vi "Practica_3.vi"() -> ()   [LabVIEW 2022 SP3]
uses:
  <vilib>/Utility/NIReport.llb/Report Type.ctl
  <vilib>/imath/engines/lvmath2/RunTimeEngine/Managers/WorkSpace/UID Generator.vi
  <vilib>/imath/engines/lvmath2/RunTimeEngine/RunTimeType/NIMS_RunTimeType_From StrictType (excl LVString).vi
  <instcachedir>/0/NIMS_RunTimeType_From StrictType (excl LVString)_70DEE8F51B6B495C85F505DE4E7061F1.lvgen/NIMS_RunTimeType_From StrictType (excl LVString)_70DEE8F51B6B495C85F505DE4E7061F1_000.vi
  <vilib>/imath/engines/lvmath2/RunTimeEngine/LocalVariableDefStatement/MC_LocalVariableDefStatement_Display.vi
  <vilib>/imath/engines/lvmath2/RunTimeEngine/VariableToken/NIMS_VariableToken_CondDefined.vi
  <instcachedir>/0/NIMS_VariableToken_CondDefined_190C34D11DD44198A50DB545329B6163.lvgen/NIMS_VariableToken_CondDefined_190C34D11DD44198A50DB545329B6163_003.vi
  <vilib>/imath/engines/lvmath2/RunTimeEngine/BuiltInFunctions/tf_to_ss/NIMS_tf_to_ss.vi
  <vilib>/imath/engines/lvmath2/RunTimeEngine/ErrorHandling/NIMS_Create Error From Enums.vi
  <vilib>/imath/engines/lvmath2/RunTimeEngine/BuiltInFunctions/transpose/NIMS_transpose(GM).vi
  <instcachedir>/0/NIMS_transpose(GM)_822C4B39CC3F4B34B360A85316D387F1.lvgen/NIMS_transpose(GM)_822C4B39CC3F4B34B360A85316D387F1_004.vi
  <vilib>/imath/engines/lvmath/Plug In/Control Design/BuiltInFunctions/obsvmx/NIMS_CD_obsvmx(A,B).vi
  <vilib>/imath/engines/lvmath/Plug In/Control Design/BuiltInFunctions/ctrbmx/NIMS_CD_ctrbmx(A,B).vi
  <vilib>/imath/engines/lvmath2/RunTimeEngine/BuiltInFunctions/rank/NIMS_rank.vi
  <instcachedir>/0/NIMS_rank_39A1B4AED7134F5694149EE328E336E6.lvgen/NIMS_rank_39A1B4AED7134F5694149EE328E336E6_000.vi
  <vilib>/imath/engines/lvmath2/RunTimeEngine/ErrorHandling/NIMS_Error From Error Code.vi
  <vilib>/imath/engines/lvmath2/RunTimeEngine/BuiltInFunctions/det/NIMS_det.vi
  <instcachedir>/0/NIMS_det_FC43403F6A814B2FA6A2876A6DC65E99.lvgen/NIMS_det_FC43403F6A814B2FA6A2876A6DC65E99_000.vi
  <vilib>/imath/engines/lvmath/Plug In/Control Design/BuiltInFunctions/ss/NIMS_CD_ss(A,B,C,D).vi
  <instcachedir>/0/NIMS_RunTimeType_From StrictType (excl LVString)_70DEE8F51B6B495C85F505DE4E7061F1.lvgen/NIMS_RunTimeType_From StrictType (excl LVString)_70DEE8F51B6B495C85F505DE4E7061F1_032.vi
  <vilib>/imath/engines/lvmath/Plug In/Control Design/BuiltInFunctions/step/NIMS_CD_[Y,T,X]=step(SS,[Tinfo]).vi
  <vilib>/imath/engines/lvmath2/RunTimeEngine/BuiltInFunctions/inv/NIMS_inv(GM).vi
  <instcachedir>/0/NIMS_inv(GM)_A6DF8FE880224208AACFE4CF9F659502.lvgen/NIMS_inv(GM)_A6DF8FE880224208AACFE4CF9F659502_000.vi
  <vilib>/imath/engines/lvmath2/RunTimeEngine/BuiltInFunctions/size/NIMS_I32Row=size(GM).vi
  <instcachedir>/0/NIMS_I32Row=size(GM)_10ACDCB9F1F84A7E9F42C91D87611FB5.lvgen/NIMS_I32Row=size(GM)_10ACDCB9F1F84A7E9F42C91D87611FB5_001.vi
  <vilib>/imath/engines/lvmath2/RunTimeEngine/IndexRead/NIMS V(S).vi
  <instcachedir>/0/NIMS V(S)_0488751826AF41519A22953C041130DC.lvgen/NIMS V(S)_0488751826AF41519A22953C041130DC_002.vi
  <vilib>/imathl/engines/lvmath/Functions/Error Handling/Create Error.vi
  <instcachedir>/0/NIMS_VariableToken_CondDefined_190C34D11DD44198A50DB545329B6163.lvgen/NIMS_VariableToken_CondDefined_190C34D11DD44198A50DB545329B6163_001.vi
  <instcachedir>/0/NIMS_VariableToken_CondDefined_190C34D11DD44198A50DB545329B6163.lvgen/NIMS_VariableToken_CondDefined_190C34D11DD44198A50DB545329B6163_005.vi
  <instcachedir>/0/NIMS_VariableToken_CondDefined_190C34D11DD44198A50DB545329B6163.lvgen/NIMS_VariableToken_CondDefined_190C34D11DD44198A50DB545329B6163_004.vi
  <vilib>/imath/engines/lvmath/Functions/Error Handling/MergeErrorsWrapper.vi
  <vilib>/imath/engines/lvmath2/RunTimeEngine/Managers/SymbolTable/Clear UID.vi
  <vilib>/imath/engines/lvmath2/RunTimeEngine/NodeEndStatement/NIMS_NodeEndStatement_Output.vi
  <instcachedir>/0/NIMS_NodeEndStatement_Output_53EC0D466D134D7ABD903AC30B43404B.lvgen/NIMS_NodeEndStatement_Output_53EC0D466D134D7ABD903AC30B43404B_009.vi
  <instcachedir>/0/NIMS_NodeEndStatement_Output_53EC0D466D134D7ABD903AC30B43404B.lvgen/NIMS_NodeEndStatement_Output_53EC0D466D134D7ABD903AC30B43404B_002.vi
  <instcachedir>/0/NIMS_NodeEndStatement_Output_53EC0D466D134D7ABD903AC30B43404B.lvgen/NIMS_NodeEndStatement_Output_53EC0D466D134D7ABD903AC30B43404B_001.vi
  <vilib>/imath/engines/lvmath2/RunTimeEngine/ErrorHandling/NIMS_Finalize Error.vi
  <vilib>/imath/engines/lvmath2/RunTimeEngine/BuiltInFunctions/sin/NIMS_sin(C).vi
  <instcachedir>/0/NIMS_sin(C)_E954A9BB68A349B3841053E554BADAA4.lvgen/NIMS_sin(C)_E954A9BB68A349B3841053E554BADAA4_001.vi
  <vilib>/imath/engines/lvmath2/RunTimeEngine/BuiltInFunctions/cos/NIMS_cos(C).vi
  <instcachedir>/0/NIMS_cos(C)_24E28D29219C4DC6ABC084DC6A0254BF.lvgen/NIMS_cos(C)_24E28D29219C4DC6ABC084DC6A0254BF_001.vi
  <vilib>/imath/engines/lvmath2/RunTimeEngine/BuiltInFunctions/length/NIMS_length(GM).vi
  <instcachedir>/0/NIMS_length(GM)_47CEC356FCE0482D9BA47DC61C99F2C7.lvgen/NIMS_length(GM)_47CEC356FCE0482D9BA47DC61C99F2C7_000.vi
  <vilib>/imath/engines/lvmath2/RunTimeEngine/BuiltInFunctions/zeros/NIMS_V=zeros(I32,I32).vi
  <vilib>/imath/engines/lvmath2/RunTimeEngine/RowToken/NIMS_RowToken_M_M.vi
  <instcachedir>/0/NIMS_RowToken_M_M_4BA134D7580D4B93A915AC56DC6FEFD1.lvgen/NIMS_RowToken_M_M_4BA134D7580D4B93A915AC56DC6FEFD1_004.vi
  <vilib>/imath/engines/lvmath2/RunTimeEngine/MatrixToken/NIMS_MatrixToken_M_RV.vi
  <instcachedir>/0/NIMS_MatrixToken_M_RV_FA177D3434DD41A3B3A5813DE937EEA2.lvgen/NIMS_MatrixToken_M_RV_FA177D3434DD41A3B3A5813DE937EEA2_001.vi
  <vilib>/imath/engines/lvmath/Plug In/Control Design/BuiltInFunctions/ackermann/NIMS_CD_ackermann(A,B,poles,STR).vi
  <vilib>/imath/engines/lvmath2/RunTimeEngine/BuiltInFunctions/eye/NIMS_M=eye(I32).vi
  <vilib>/imath/engines/lvmath2/RunTimeEngine/ArithmeticOperatorToken/NIMS_ArithmeticOperator_minus.vi
  <instcachedir>/0/NIMS_ArithmeticOperator_minus_22EE3FD1C8824638A4ED1C446A3DB56D.lvgen/NIMS_ArithmeticOperator_minus_22EE3FD1C8824638A4ED1C446A3DB56D_001.vi
  <vilib>/imath/engines/lvmath2/RunTimeEngine/ArithmeticOperatorToken/NIMS_ArithmeticOperator_plus.vi
  <instcachedir>/0/NIMS_ArithmeticOperator_plus_3E2F46F6B6A2434E909AF418D4802C21.lvgen/NIMS_ArithmeticOperator_plus_3E2F46F6B6A2434E909AF418D4802C21_011.vi
  <vilib>/imath/engines/lvmath2/RunTimeEngine/ArithmeticOperatorToken/NIMS_ArithmeticOperator_multmx.vi
  <instcachedir>/0/NIMS_ArithmeticOperator_multmx_BDE1B5075EB4429787EED704427CBD98.lvgen/NIMS_ArithmeticOperator_multmx_BDE1B5075EB4429787EED704427CBD98_004.vi
  <vilib>/imath/engines/lvmath2/RunTimeEngine/MatrixToken/NIMS_MatrixToken_M_M.vi
  <instcachedir>/0/NIMS_MatrixToken_M_M_35B6F7FCE524444C982F4243CAF19F60.lvgen/NIMS_MatrixToken_M_M_35B6F7FCE524444C982F4243CAF19F60_004.vi
  <vilib>/imath/engines/lvmath2/RunTimeEngine/ArithmeticOperatorToken/NIMS_ArithmeticOperator_multmx(RV,M).vi
  <instcachedir>/0/NIMS_ArithmeticOperator_multmx(RV,M)_0C5EC56C64A44F5D9A149E640905A95E.lvgen/NIMS_ArithmeticOperator_multmx(RV,M)_0C5EC56C64A44F5D9A149E640905A95E_001.vi
  <vilib>/imath/engines/lvmath2/RunTimeEngine/IndexRead/NIMS M(R2).vi
  <instcachedir>/0/NIMS M(R2)_287818D58BD74005B29FE73CE7602B1A.lvgen/NIMS M(R2)_287818D58BD74005B29FE73CE7602B1A_000.vi
  <vilib>/imath/engines/lvmath2/RunTimeEngine/IndexRead/NIMS M(V).vi
  <instcachedir>/0/NIMS M(V)_948FAC22C1C943948B75DA6190348614.lvgen/NIMS M(V)_948FAC22C1C943948B75DA6190348614_005.vi
  <instcachedir>/0/NIMS_NodeEndStatement_Output_53EC0D466D134D7ABD903AC30B43404B.lvgen/NIMS_NodeEndStatement_Output_53EC0D466D134D7ABD903AC30B43404B_005.vi
  <instcachedir>/0/NIMS_NodeEndStatement_Output_53EC0D466D134D7ABD903AC30B43404B.lvgen/NIMS_NodeEndStatement_Output_53EC0D466D134D7ABD903AC30B43404B_008.vi
  <vilib>/imath/engines/lvmath2/RunTimeEngine/IndexRead/NIMS V($).vi
  <instcachedir>/0/NIMS V($)_C593F32C7F6B43C7B1793952E292524F.lvgen/NIMS V($)_C593F32C7F6B43C7B1793952E292524F_001.vi
  <vilib>/imath/engines/lvmath2/RunTimeEngine/ArithmeticOperatorToken/NIMS_ArithmeticOperator_multmx(M,CV).vi
  <instcachedir>/0/NIMS_ArithmeticOperator_multmx(M,CV)_F5DBFFF0126A4383B39F7B34D5ABA6C8.lvgen/NIMS_ArithmeticOperator_multmx(M,CV)_F5DBFFF0126A4383B39F7B34D5ABA6C8_000.vi
  <instcachedir>/0/NIMS_ArithmeticOperator_minus_22EE3FD1C8824638A4ED1C446A3DB56D.lvgen/NIMS_ArithmeticOperator_minus_22EE3FD1C8824638A4ED1C446A3DB56D_002.vi
  <vilib>/imath/engines/lvmath2/RunTimeEngine/IndexRead/NIMS M(S,S).vi
  <instcachedir>/0/NIMS M(S,S)_AC51E74150A542F7991B9634C66F3096.lvgen/NIMS M(S,S)_AC51E74150A542F7991B9634C66F3096_000.vi
  <vilib>/imath/engines/lvmath2/RunTimeEngine/IndexRead/NIMS M($).vi
  <instcachedir>/0/NIMS M($)_82D1177398184AFB96A6AFB63C3C3F57.lvgen/NIMS M($)_82D1177398184AFB96A6AFB63C3C3F57_000.vi
  <instcachedir>/0/NIMS_ArithmeticOperator_plus_3E2F46F6B6A2434E909AF418D4802C21.lvgen/NIMS_ArithmeticOperator_plus_3E2F46F6B6A2434E909AF418D4802C21_003.vi
  <vilib>/addons/_office/excel.llb/Excel Easy Table (num).vi
  <vilib>/Utility/NIReport.llb/NI_report.lvclass
  <vilib>/imath/engines/lvmath2/RunTimeEngine/Managers/SymbolTable/NIMS_WorkSpace.lvlib
  <vilib>/addons/_office/NI_ReportGenerationToolkit.lvlib
  <vilib>/Utility/NIReport.llb/Excel/NI_Excel.lvclass
  <vilib>/Utility/NIReport.llb/NI_ReportGenerationCore.lvlib
panel:
  out "xk1":dbl[](array[numeric])
  out "yk 2":dbl
  out "salida controlada":dbl
  out "set point":dbl
  in  "Tab Control":T1(tab)
  out "Observabilidad":string="El Sistema es Controlabe"
  out "Controlabilidas":string="El Sistema es Controlabe"
  out "Ta_Mo":i32
  out "Ta_Mc":i32
  out "GRAFICA":dbl[][](graph)
  out "Dete_MO":dbl
  out "Dete_MC":dbl
  out "Rango_MO":i32
  out "Rango_MC":i32
  out "MC":dbl[][](array[numeric])
  out "MO":dbl[][](array[numeric])
  out "CO":dbl[][](array[numeric])
  out "BO":dbl[][](array[numeric])
  out "AO":dbl[][](array[numeric])
  out "C":dbl[][](array[numeric])
  out "B":dbl[][](array[numeric])
  out "A":dbl[][](array[numeric])
  in  "ORDEN":dbl
  in  "Stop":bool
  in  "b4":dbl
  in  "a4":dbl
  in  "b3":dbl
  in  "a2":dbl
  in  "b2":dbl
  in  "b1":dbl
  in  "b0":dbl
  in  "a1":dbl
  in  "a3":dbl
  in  "tso":dbl
  in  "T":dbl
  in  "tss":dbl
  in  "Fa":dbl
  out "p1_o":cdb
  out "p2_o":cdb
  out "p1":cdb
  out "p2":cdb
  out "Ki":dbl[][](array[numeric])
  out "ks":dbl[][](array[numeric])
  out "L":dbl[](array[numeric])
  out "k1":dbl[][](array[numeric])
  in  "Sp":dbl
  out "Waveform Chart":T2(graph)
  out "error":dbl
  out "ley de control":dbl
  out "yk":dbl
  in  "template (empty)":path
  out "K":dbl[](array[numeric])
  out "0bservador":dbl
  # "z^-1  +"
  # "z^-2  +"
  # "z^-3  +"
  # "z^-4"
  # "+"
  # "Y(z)"
  # "G(Z)="
  # "="
  # "U(z)"
  # "z^-1  +"
  # "z^-2  +"
  # "z^-3  +"
  # "z^-4"
  # "1  +"
  # "FORMA CANONICA CONTROLABLE"
  # "FORMA CANONICA OBSERVABLE"
  # "CONTROLABILIDAD Y OBSERVABILIDAD DEL SISTEMA"
  # "CONDICIONES DE DISEÑO"
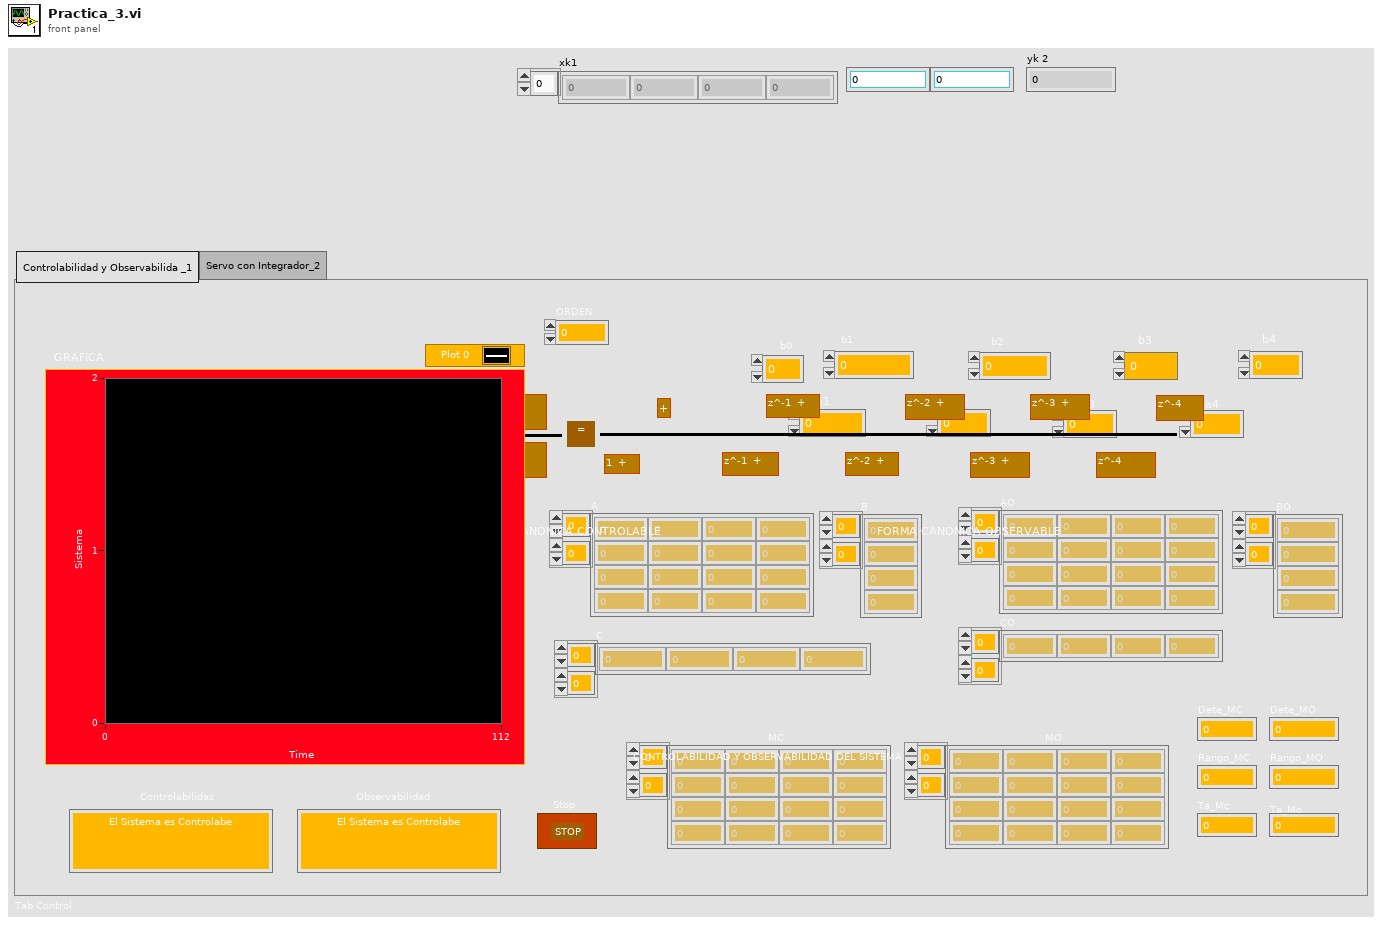
[diagram p1: front panel]
types:
  T1 = enum32{"Controlabilidad y Observabilida _1", "Servo con Integrador_2"}
  T2 = cluster{"yk":dbl, "Set-point":dbl, "error":dbl, dbl, dbl}
  T3 = typedef "NI_ReportGenerationCore.lvlib/Report Type.ctl" = enum16{"HTML", "Word", "Excel"}
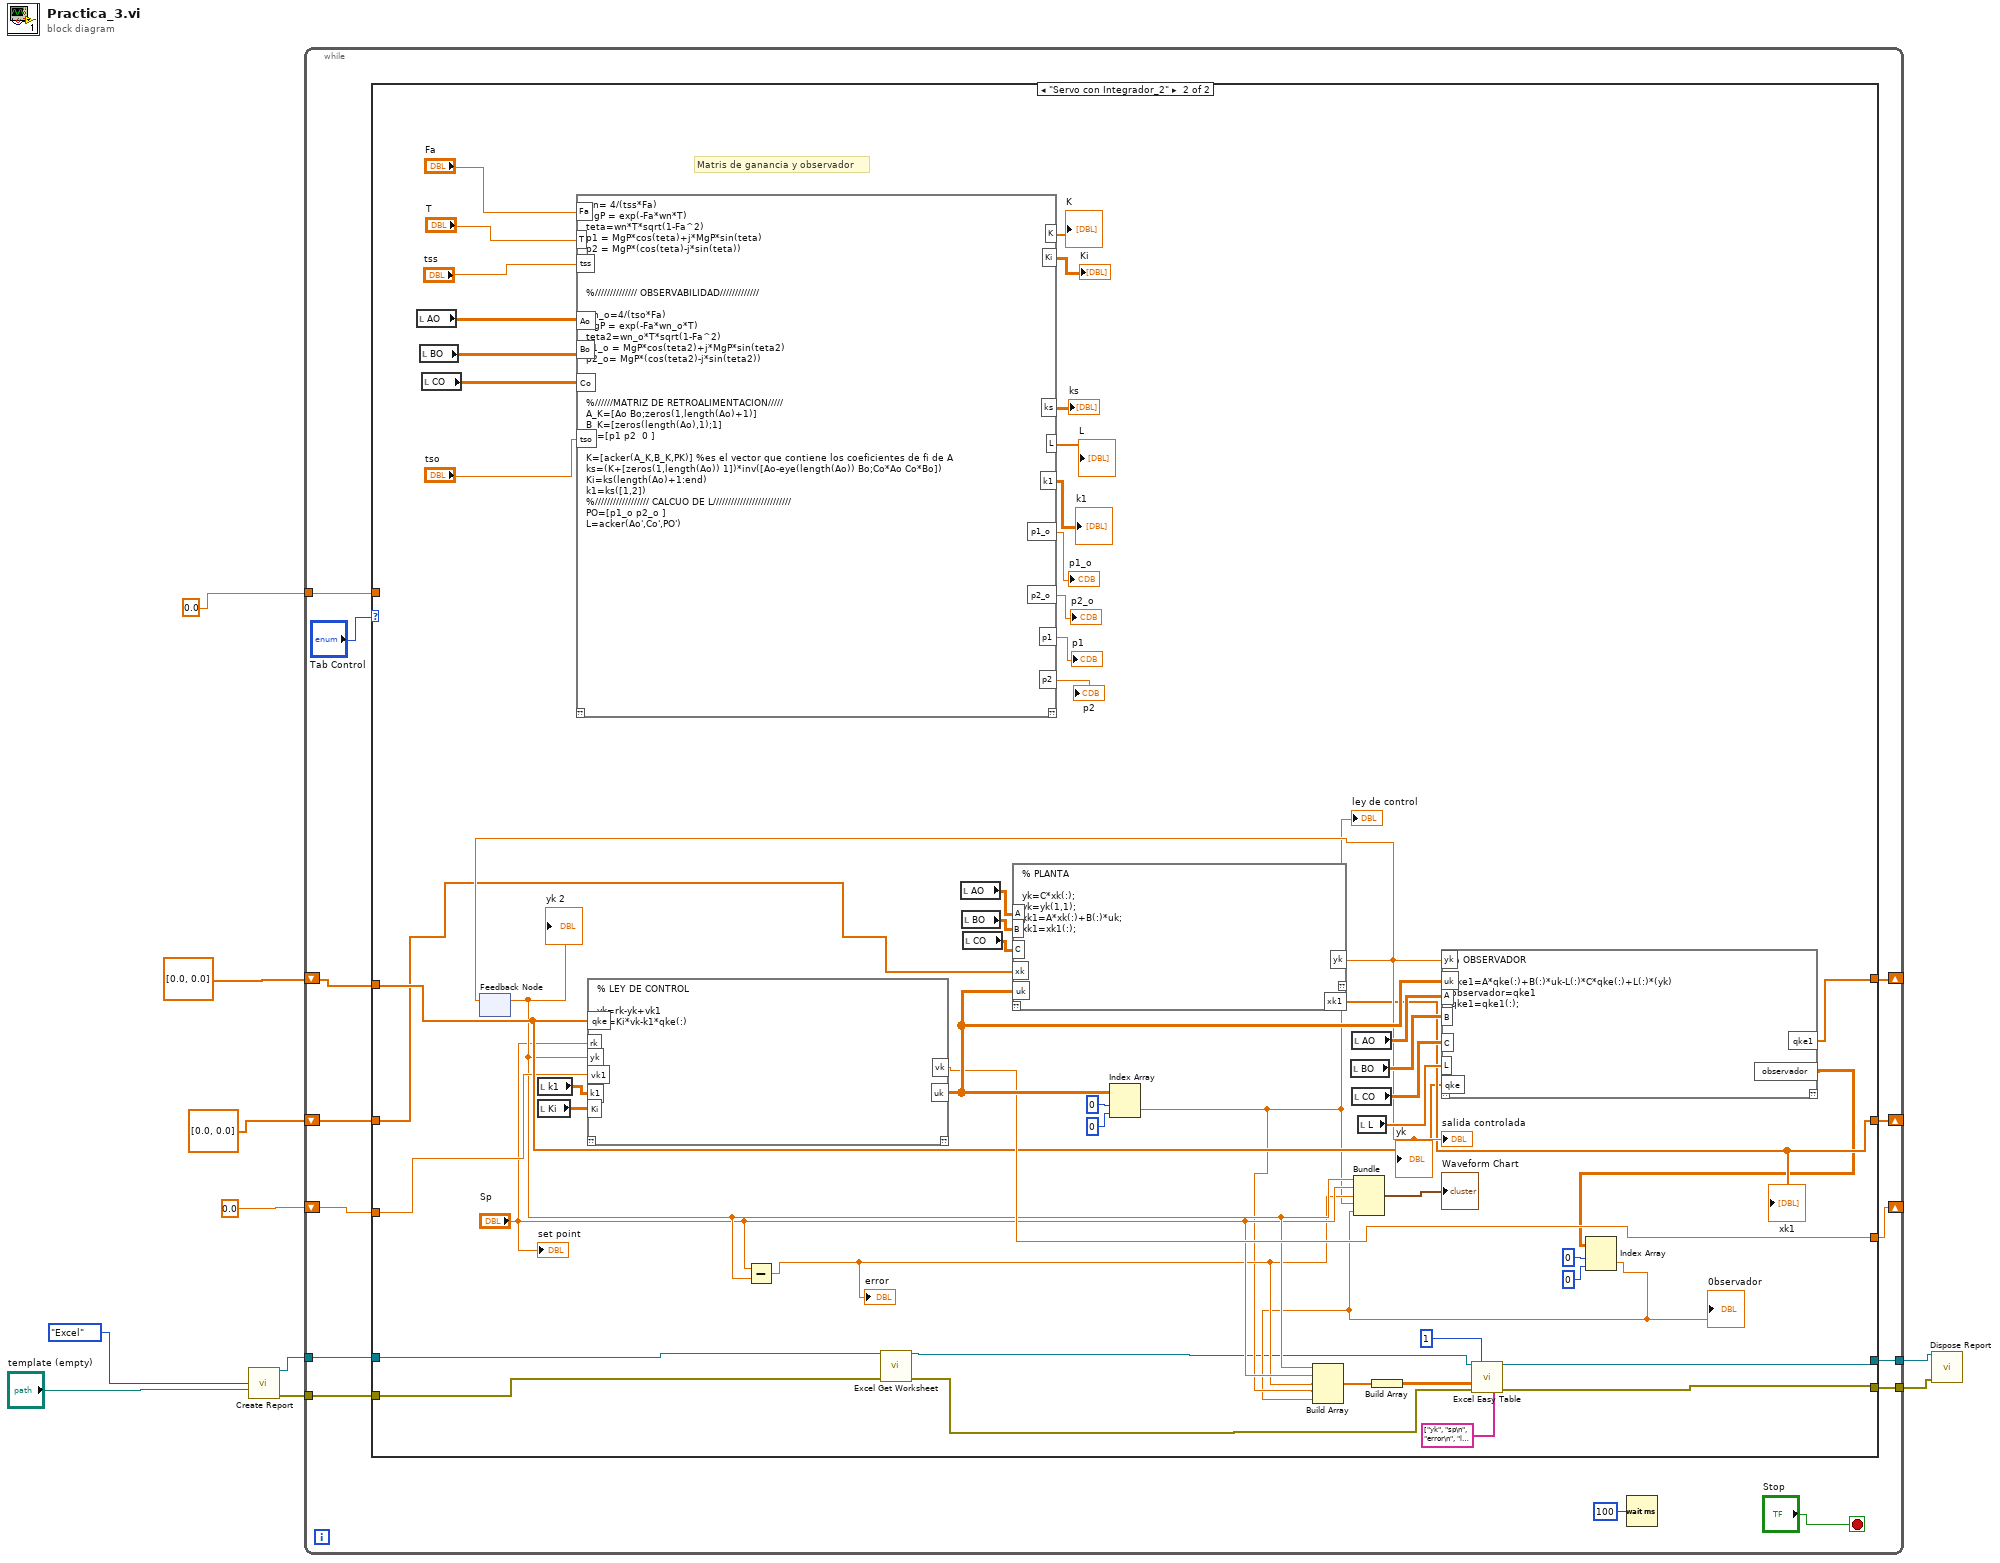
[diagram p0: block diagram]
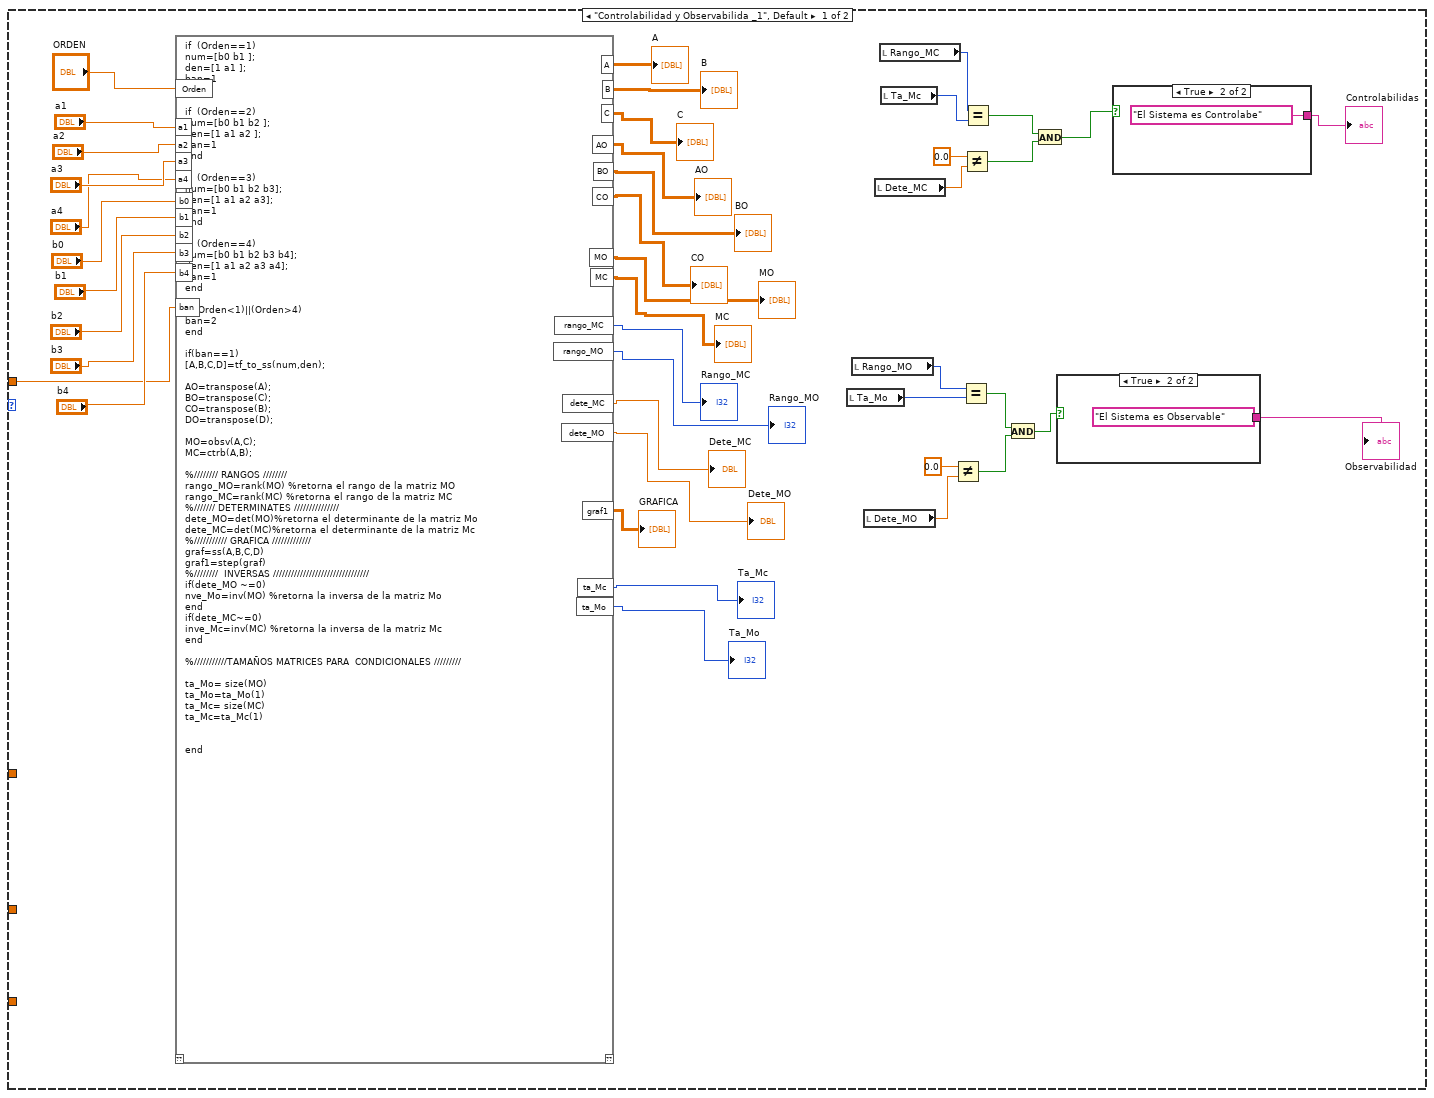
[diagram p2: hidden frame]
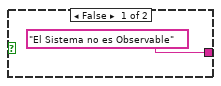
[diagram p3: hidden frame]
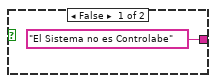
[diagram p4: hidden frame]
diagram:
  n1 = call <vilib>:"Create Report.vi"("report type"=Report_Type."Excel", "template (empty)"="template (empty)") -> ("report out"=w2:refnum<class "NI_report.lvclass">, "error out"=w1:errorcluster)  [unwired: 12 in]
  n2 = while {
    tunnel: 0.0 ("ban") -> [w22]
    shift-right: [w20] -> _
    shift-left: dbl[] [0.0, 0.0] ("qke1") -> [w19]
    shift-right: [w18] -> _
    shift-left: dbl[] [0.0, 0.0] ("xk1") -> [w17]
    shift-right: [w16] -> _
    shift-left: 0.0 ("yk") -> [w15]
    tunnel: [w14] -> w6
    tunnel: [w13] -> w5
    tunnel: w2 -> [w12]
    tunnel: w1 -> [w11]
    stop <- "Stop" stop-if-true
    n3 = case shown="\"Servo con Integrador_2\"" "Tab Control" {
      tunnel: w22 -> [w56 _]
      tunnel: [_ w1020] -> w20
      tunnel: w19 -> [_ w1016]
      tunnel: [_ w1019] -> w18
      tunnel: w17 -> [_ w1014]
      tunnel: [_ w1018] -> w16
      tunnel: w15 -> [_ w1015]
      tunnel: [_ w1002] -> w14
      tunnel: [_ w1001] -> w13
      tunnel: w12 -> [_ w1000]
      tunnel: w11 -> [_ w999]
      frame "Controlabilidad y Observabilida _1", Default {
        n4 = mathscript code="if  (Orden==1)\nnum=[b0 b1 ];\nden=[1 a1 ];\nban=1\nend \n\nif  (Orden==2)\nnum=[b0 b1 b2 ];\nden=[1 a1 a2 ];\nban=1\nend \n\nif  (Orden==3)\nnum=[b0 b1 b2 b3];\nden=[1 a1 a2 a3];\nban=1\nend \n\nif  (Orden==4)\nnum=[b0 b1 b2 b3 b4];\nden=[1 a1 a2 a3 a4];\nban=1\nend \n\nif (Orden<1)||(Orden>4)\nban=2\nend\n\nif(ban==1) \n[A,B,C,D]=tf_to_ss(num,den);\n\nAO=transpose(A);\nBO=transpose(C);\nCO=transpose(B);\nDO=transpose(D);\n\nMO=obsv(A,C);\nMC=ctrb(A,B);\n\n%//////// RANGOS ////////\nrango_MO=rank(MO) %retorna el rango de la matriz MO\nrango_MC=rank(MC) %retorna el rango de la matriz MC\n%/////// DETERMINATES ///////////////\ndete_MO=det(MO)%retorna el determinante de la matriz Mo\ndete_MC=det(MC)%retorna el determinante de la matriz Mc\n%/////////// GRAFICA /////////////\ngraf=ss(A,B,C,D)\ngraf1=step(graf)\n%////////  INVERSAS ////////////////////////////////\nif(dete_MO ~=0)\nnve_Mo=inv(MO) %retorna la inversa de la matriz Mo\nend\nif(dete_MC~=0)\ninve_Mc=inv(MC) %retorna la inversa de la matriz Mc\nend\n\n%///////////TAMAÑOS MATRICES PARA  CONDICIONALES /////////\n\nta_Mo= size(MO)\nta_Mo=ta_Mo(1)\nta_Mc= size(MC)\nta_Mc=ta_Mc(1)\n\n \nend"("a1"="a1", "a2"="a2", "a3"="a3", "a4"="a4", "b0"="b0", "b1"="b1", "b2"="b2", "b3"="b3", "b4"="b4", "Orden"="ORDEN", "ban"=w56) -> ("A"=→"A":dbl[][], "B"=→"B":dbl[][], "C"=→"C":dbl[][], "AO"=→"AO":dbl[][], "BO"=→"BO":dbl[][], "CO"=→"CO":dbl[][], "MO"=→"MO":dbl[][], "MC"=→"MC":dbl[][], "rango_MC"=→"Rango_MC":i32, "rango_MO"=→"Rango_MO":i32, "dete_MC"=→"Dete_MC":dbl, "dete_MO"=→"Dete_MO":dbl, "graf1"=→"GRAFICA":dbl[][], "ta_Mc"=→"Ta_Mc":i32, "ta_Mo"=→"Ta_Mo":i32)  [unwired: 1 in, 1 out]
        n5 = local read "Ta_Mo"() -> (w25:i32)
        n6 = local read "Rango_MO"() -> (w26:i32)
        n7 = local read "Dete_MO"() -> (w27:dbl)
        n8 = local read "Dete_MC"() -> (w33:dbl)
        n9 = local read "Rango_MC"() -> (w36:i32)
        n10 = local read "Ta_Mc"() -> (w35:i32)
        n11 = Not Equal?(x=0.0, y=w27) -> (x != y?=w30:bool)
        n12 = Equal?(x=w26, y=w25) -> (x = y?=w31:bool)
        n13 = Not Equal?(x=0.0, y=w33) -> (x != y?=w38:bool)
        n14 = Equal?(x=w36, y=w35) -> (x = y?=w40:bool)
        n15 = And(x=w31, y=w30) -> (x .and. y?=w29:bool)
        n16 = And(x=w40, y=w38) -> (x .and. y?=w39:bool)
        n17 = case shown="True" w29 {
          tunnel: ["El Sistema no es Observable" "El Sistema es Observable"] -> w28
          frame False {
          }
          frame True {
          }
        }
        "Observabilidad" <- w28
        n18 = case shown="True" w39 {
          tunnel: ["El Sistema no es Controlabe" "El Sistema es Controlabe"] -> w37
          frame False {
          }
          frame True {
          }
        }
        "Controlabilidas" <- w37
      }
      frame "Servo con Integrador_2" {
        # "Matris de ganancia y observador"
        n19 = local read "AO"() -> (w1047:dbl[][])
        n20 = local read "BO"() -> (w1046:dbl[][])
        n21 = local read "CO"() -> (w1045:dbl[][])
        n22 = feedback #1() -> (w1011:dbl)  [unwired: 1 in]
        "yk 2" <- w1011
        n23 = local read "k1"() -> (w1032:dbl[][])
        n24 = local read "Ki"() -> (w1033:dbl[][])
        n25 = mathscript code="wn= 4/(tss*Fa)\nMgP = exp(-Fa*wn*T)\nteta=wn*T*sqrt(1-Fa^2)\np1 = MgP*cos(teta)+j*MgP*sin(teta)\np2 = MgP*(cos(teta)-j*sin(teta))\n\n\n\n%////////////// OBSERVABILIDAD/////////////\n\nwn_o=4/(tso*Fa)\nMgP = exp(-Fa*wn_o*T)\nteta2=wn_o*T*sqrt(1-Fa^2)\np1_o = MgP*cos(teta2)+j*MgP*sin(teta2)\np2_o= MgP*(cos(teta2)-j*sin(teta2))\n\n\n\n%//////MATRIZ DE RETROALIMENTACION/////\nA_K=[Ao Bo;zeros(1,length(Ao)+1)]\nB_K=[zeros(length(Ao),1);1]\nPK=[p1 p2  0 ]\n\nK=[acker(A_K,B_K,PK)] %es el vector que contiene los coeficientes de fi de A\nks=(K+[zeros(1,length(Ao)) 1])*inv([Ao-eye(length(Ao)) Bo;Co*Ao Co*Bo])\nKi=ks(length(Ao)+1:end)\nk1=ks([1,2])\n%////////////////// CALCUO DE L//////////////////////////\nPO=[p1_o p2_o ]\nL=acker(Ao',Co',PO')"("Fa"="Fa", "T"="T", "tss"="tss", "Ao"=w1047, "Bo"=w1046, "Co"=w1045, "tso"="tso") -> ("K"=→"K":dbl[], "Ki"=→"Ki":dbl[][], "ks"=→"ks":dbl[][], "p1_o"=→"p1_o":cdb, "p2_o"=→"p2_o":cdb, "p1"=→"p1":cdb, "p2"=→"p2":cdb, "L"=→"L":dbl[], "k1"=→"k1":dbl[][])  [unwired: 1 in, 1 out]
        n26 = mathscript code="% LEY DE CONTROL \n\nvk=rk-yk+vk1\nuk=Ki*vk-k1*qke(:)"("rk"="Sp", "yk"=w1011, "vk1"=w1015, "k1"=w1032, "Ki"=w1033, "qke"=w1016) -> ("vk"=w1018:dbl, "uk"=w1024:dbl[][])  [unwired: 1 in, 1 out]
        n27 = Subtract(x="Sp", y=w1011) -> (x-y=w1009:dbl)
        "error" <- w1009
        n28 = call <vilib>:"Excel Get Worksheet.vi"("report in"=w1000, "error in (no error)"=w999) -> ("report out"=w1003:refnum<class "NI_report.lvclass">, "error out"=w1004:errorcluster)  [unwired: 12 in]
        n29 = local read "AO"() -> (w1036:dbl[][])
        n30 = local read "BO"() -> (w1035:dbl[][])
        n31 = local read "CO"() -> (w1034:dbl[][])
        n32 = mathscript code="% PLANTA \n\nyk=C*xk(:);\nyk=yk(1,1); \nxk1=A*xk(:)+B(:)*uk;\nxk1=xk1(:);"("A"=w1036, "B"=w1035, "C"=w1034, "xk"=w1014, "uk"=w1024) -> ("xk1"=w1019:dbl[], "yk"=w1023:dbl)  [unwired: 1 in, 1 out]
        "salida controlada" <- w1023
        "yk" <- w1023
        "xk1" <- w1019
        n33 = feedback-in #1(w1023) -> ()
        n34 = Index Array(array=w1024, index (row)=0 ("disabled index (row)"), index (col)=0 ("disabled index (col)")) -> (element=w1008:dbl)
        "ley de control" <- w1008
        n35 = local read "BO"() -> (w1026:dbl[][])
        n36 = local read "AO"() -> (w1025:dbl[][])
        n37 = local read "CO"() -> (w1027:dbl[][])
        n38 = local read "L"() -> (w1028:dbl[])
        n39 = mathscript code="% OBSERVADOR\n\nqke1=A*qke(:)+B(:)*uk-L(:)*C*qke(:)+L(:)*(yk)\nobservador=qke1\nqke1=qke1(:);"("A"=w1025, "B"=w1026, "C"=w1027, "L"=w1028, "qke"=w1016, "uk"=w1024, "yk"=w1023) -> ("qke1"=w1020:dbl[], "observador"=w1017:dbl[][])  [unwired: 1 in, 1 out]
        n40 = Index Array(array=w1017, index (row)=0 ("disabled index (row)"), index (col)=0 ("disabled index (col)")) -> (element=w1007:dbl)
        "0bservador" <- w1007
        n41 = Build Array(w1011, "Sp", w1009, w1008, w1007) -> (w1006:dbl[])
        n42 = Bundle("yk"=w1011, "Sp"="Sp", w1009, w1008, w1007) -> (→"Waveform Chart":cluster{"yk":dbl, "Sp\n":dbl, dbl, dbl, dbl})  [unwired: 1 in]
        n43 = Build Array(w1006) -> (w1013:dbl[][])
        n44 = call-poly <vilib>:"Excel Easy Table.vi"("report in"=w1003, "iteration"=1, "text data"=w1013, "error in (no error)"=w1004, "column headers"=string[] ["yk", "sp\n", "error\n", "ley c\n", "ob\n"]) -> ("report out"=w1002:refnum<class "NI_report.lvclass">, "error out"=w1001:errorcluster)  [unwired: 6 in, 3 out]
        "set point" <- "Sp"
      }
    }
    n45 = Wait (ms)(milliseconds to wait=u32 100) -> ()  [unwired: 1 out]
  }
  n46 = call-dynamic "Dispose Report.vi"("report in"=w6, "error in (no error)"=w5) -> ()  [unwired: 13 in, 1 out]
